vi "InitPacket.vi"() -> (3 "string":string)   [LabVIEW 2018]
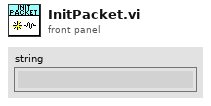
[diagram p1: front panel]
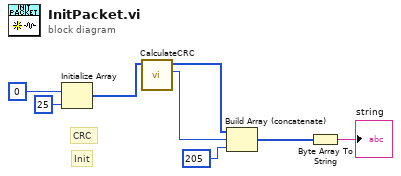
[diagram p0: block diagram]
diagram:
  # "Init"
  # "CRC"
  n1 = Initialize Array(u8 0, 25 ("dimension size")) -> (w5:u8[])
  n2 = call "CalculateCRC.vi"("data in"=w5) -> ("CRC"=w7:u8, "data out"=w6:u8[])  [unwired: 9 in]
  n3 = Build Array (concatenate)(w6, w7, u8 205) -> (w3:u8[])
  n4 = Byte Array To String(unsigned byte array=w3) -> (string=→"string":string)
